vi "ATF-Sample Rate Ring Update.vi"(10 "SR":u16[](array[numeric]), 11 "DL":tag[](array[tag])) -> (3 "Array":string[][](array[string]))   [LabVIEW 2022 SP3]
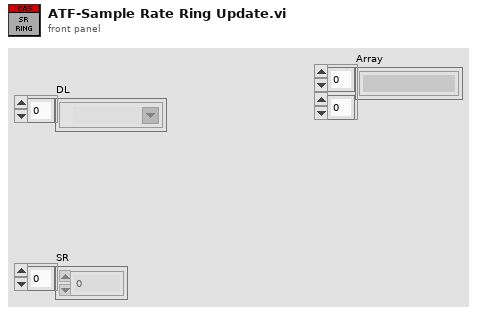
[diagram p1: front panel]
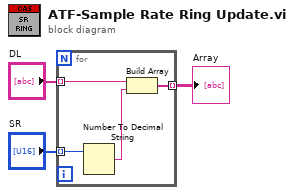
[diagram p0: block diagram]
diagram:
  n1 = for {
    tunnel: "DL" -> [w6] mode=indexing
    tunnel: "SR" -> [w7] mode=indexing
    tunnel: [w4] -> w1 mode=indexing
    n2 = Number To Decimal String(number=w7) -> (decimal integer string=w5:string)  [unwired: 1 in]
    n3 = Build Array(w6, w5) -> (w4:string[])
  }
  "Array" <- w1
